vi "Configure NCO.vi"(8 "error in (no error)":errorcluster, 10 "nco.frequency 0":fxp<+/-,48,0> format="%.48g", 11 "LIA Host Interface in":refnum<class "LIA Host Interface.lvclass">) -> (0 "error out":errorcluster, 3 "LIA Host Interface out":refnum<class "LIA Host Interface.lvclass">)   [LabVIEW 2018, in "LIA Debugging.lvclass"]
uses:
  LIA Debugging.lvclass
  Shared/lib/interface/Interface/LIA Host Interface.lvclass
  Shared/lib/interface/Interface FPGA/LIA Host Interface FPGA.lvclass
  Shared/lib/interface/Interface FPGA/Properties/FpgaSession_GET.vi
  <vilib>/Utility/error.llb/Error Cluster From Error Code.vi
  <vilib>/rvi/errors/niLvFpgaAdjustHostInterfaceError.vi
  <vilib>/rvi/interface/nirviReadWriteControl/nirviReadWriteControl.xnode
  NiFpgaLv.dll
  <vilib>/rvi/interface/Simulation/niFpgaSimulationCallBeginRW.vi
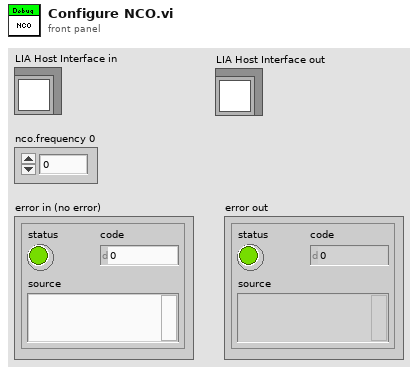
[diagram p1: front panel]
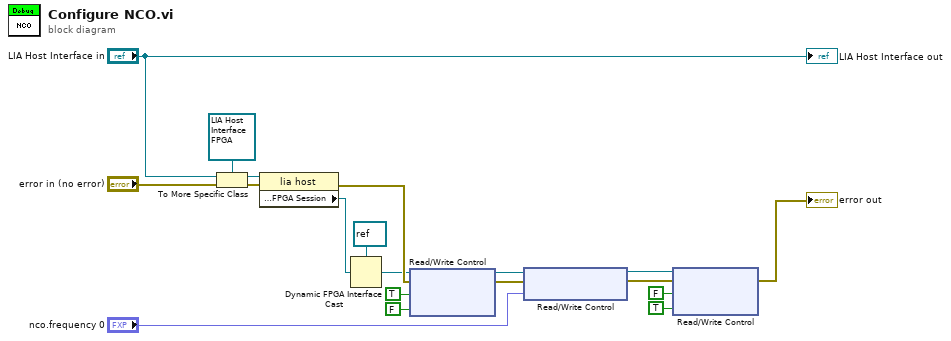
[diagram p0: block diagram]
diagram:
  n1 = To More Specific Class(target class=refnum<class "LIA Host Interface FPGA.lvclass"> refnum ("lia host"), reference="LIA Host Interface in", error in="error in (no error)") -> (specific class reference=w9:refnum<class "LIA Host Interface FPGA.lvclass">, error out=w8:errorcluster)
  n2 = property class="lia host"(reference=w9, error in=w8) -> (error out=w17:errorcluster, "Properties:FPGA Session"=w5:refnum<k20>)  [unwired: 1 out]
  n3 = Dynamic FPGA Interface Cast(Session In=refnum<k20> refnum ("fpga type"), Type=w5) -> (Session Out=w7:refnum<k20>)
  n4 = xnode "Read/Write Control"("FPGA VI Reference In"=w7, "error in"=w17, "nco.reset 0"=TRUE, "nco.enable 0"=FALSE) -> ("FPGA VI Reference Out"=w11:refnum<k20>, "error out"=w12:errorcluster)
  n5 = xnode "Read/Write Control"("FPGA VI Reference In"=w11, "error in"=w12, "nco.frequency 0"="nco.frequency 0") -> ("FPGA VI Reference Out"=w14:refnum<k20>, "error out"=w15:errorcluster)
  n6 = xnode "Read/Write Control"("FPGA VI Reference In"=w14, "error in"=w15, "nco.reset 0"=FALSE, "nco.enable 0"=TRUE) -> ("error out"=→"error out":errorcluster)  [unwired: 1 out]
  "LIA Host Interface out" <- "LIA Host Interface in"
